vi "NI VeriStand - Add Custom Device Dependencies.vi"(8 "error in (no error)":errorcluster, 10 "Dependencies":T1[](array[typedef]), 11 "Device Ref in":T5 format="%.0x") -> (0 "error out":errorcluster, 3 "Device Ref out":T5 format="%.0x")   [LabVIEW 2026, in "Custom Devices Storage.lvlib"]
uses:
  Custom Devices Storage.lvlib
  <vilib>/NI VeriStand/Custom Device API/Custom Device Item Ref.ctl
  <vilib>/NI VeriStand/Custom Device API/Custom Device API.lvlib
  <vilib>/NI VeriStand/Custom Device API/Path Type.ctl
  <vilib>/NI VeriStand/Custom Device API/Path Specification.ctl
  <vilib>/NI VeriStand/Custom Device API/Custom Device Supported Target.ctl
  <vilib>/NI VeriStand/Custom Device API/Custom Device File Dependency.ctl
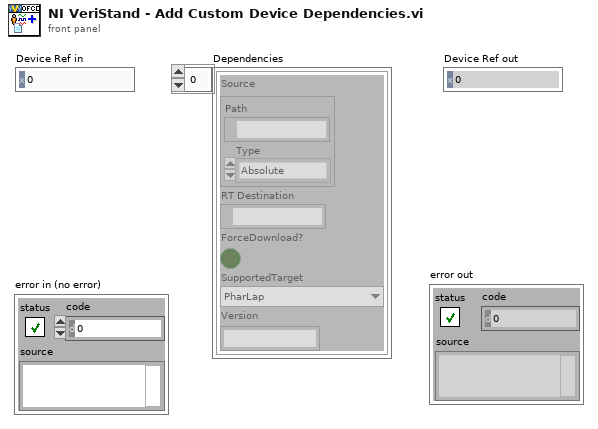
[diagram p1: front panel]
types:
  T1 = typedef "Custom Device API.lvlib/Custom Device File Dependency.ctl" = cluster{"Source":T2, "RT Destination":path, "ForceDownload?":bool, "SupportedTarget":T4, "Version":string}
  T2 = typedef "Custom Device API.lvlib/Path Specification.ctl" = cluster{"Path":path, "Type":T3}
  T3 = typedef "Custom Device API.lvlib/Path Type.ctl" = enum16{"Absolute", "To Base", "To Common Data Dir", "To Application Data Dir"}
  T4 = typedef "Custom Device API.lvlib/Custom Device Supported Target.ctl" = enum16{"All", "PharLap", "VxWorks", "Windows", "Linux_32_ARM", "Linux_x64", "PharLap & Windows", "PharLap & VxWorks", "VxWorks & Windows"}
  T5 = typedef "Custom Device API.lvlib/Custom Device Item Ref.ctl" = u64
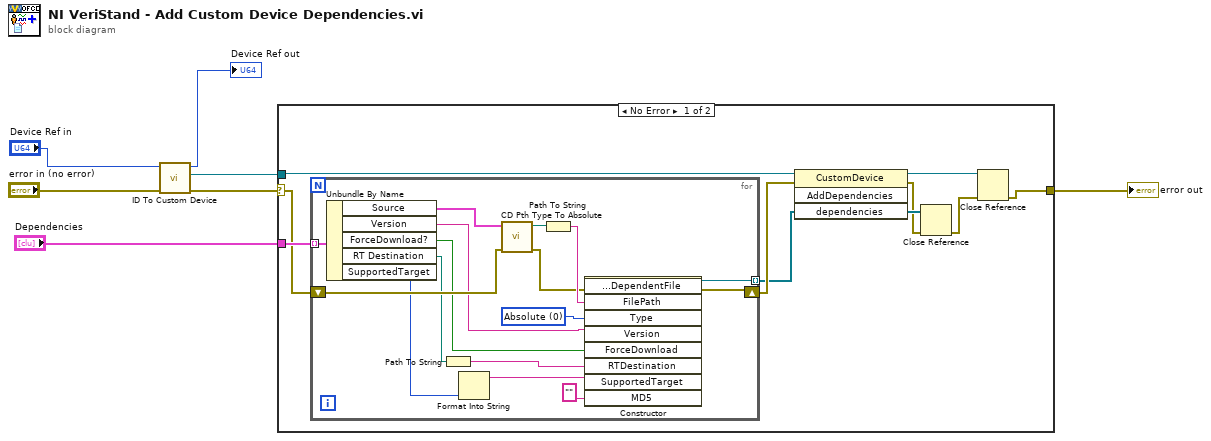
[diagram p0: block diagram]
diagram:
  n1 = call "ID To Custom Device.vi"("error in (no error)"="error in (no error)", "ID in"="Device Ref in") -> ("error out"=w5:errorcluster, "Device"=w3:refnum<k39>, "ID out"=→"Device Ref out":u64)  [unwired: 7 in]
  n2 = case shown="No Error" w5 {
    selector: w5 -> [w16 w34]
    tunnel: w3 -> [w15 _]
    tunnel: "Dependencies" -> [w17 _]
    tunnel: [w8 w34] -> w1
    frame No Error {
      n3 = for {
        tunnel: w17 -> [w33] mode=indexing
        shift-right: [w24] -> w14
        shift-left: w16 -> [w31]
        tunnel: [w23] -> w13 mode=indexing
        w28 = 0 items=["Absolute", "Relative", "ToCommonDocDir", "ToAppDataDir"] ("Type")
        n4 = Unbundle By Name(w33) -> ("Source"=w32:T2, "Version"=w19:string, "ForceDownload?"=w18:bool, "RT Destination"=w20:path, "SupportedTarget"=w21:T4)
        n5 = Path To String(path=w20) -> (string=w29:string)
        n6 = Format Into String(w21) -> (resulting string=w30:string)  [unwired: 3 in, 1 out]
        n7 = call "CD Pth Type To Absolute.vi"("error in (no error)"=w31, "CD Path Pair"=w32) -> ("error out"=w25:errorcluster, "Absolute Path"=w27:path)  [unwired: 8 in]
        n8 = Path To String(path=w27) -> (string=w26:string)
        n9 = constructor class="DependentFile"(error in=w25, "FilePath"=w26, "Type"=w28, "Version"=w19, "ForceDownload"=w18, "RTDestination"=w29, "SupportedTarget"=w30, "MD5"="" ("Version")) -> (reference out=w23:refnum<k39>, error out=w24:errorcluster)  [unwired: 2 in, 8 out]
      }
      n10 = invoke class="CustomDevice" method="AddDependencies"(reference=w15, error in=w14, "dependencies"=w13) -> (reference out=w9:refnum<k39>, error out=w11:errorcluster, "dependencies"=w12:refnum<k39>[])  [unwired: 1 in, 1 out]
      n11 = Close Reference(reference=w12, error in (no error)=w11) -> (error out=w10:errorcluster)
      n12 = Close Reference(reference=w9, error in (no error)=w10) -> (error out=w8:errorcluster)
    }
    frame Error {
    }
  }
  "error out" <- w1
